vi "Divider.vi"(0 "reset":bool, 5 "divide value":u8) -> (4 "count done":bool)   [LabVIEW 2015, in "SPI API.lvlib"]
doc: "Simple counter creates a pulse on count done everytime that the counter expires."
uses:
  SPI API.lvlib
panel:
  # "Simple counter creates a pulse on count done everytime that the counter expires."
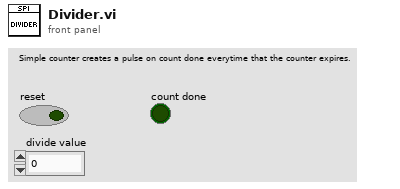
[diagram p1: front panel]
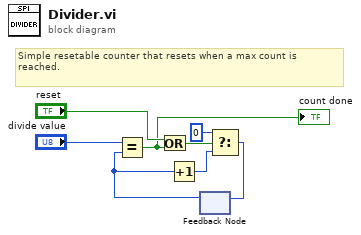
[diagram p0: block diagram]
diagram:
  # "Simple resetable counter that resets when a max count is reached."
  n1 = feedback #1() -> (w7:u8)  [unwired: 1 in]
  n2 = Equal?(x="divide value", y=w7) -> (x = y?=w1:bool)
  "count done" <- w1
  n3 = Or(x="reset", y=w1) -> (x .or. y?=w5:bool)
  n4 = Increment(x=w7) -> (x+1=w6:u8)
  n5 = Select(t=u8 0 ("DataToSend"), s=w5, f=w6) -> (s? t:f=w4:u8)
  n6 = feedback-in #1(w4) -> ()
